vi "ObjectHandler.Main.vi"() -> ()   [LabVIEW 2016, in "ObjectHandler.lvclass"]
uses:
  ObjectHandler.lvclass
  Package Libraries/Message Queue/private/MessageQueue.MessageTypeDef.ctl
  ObjectHandler.lvclass/ObjectHandler.ctl
  ObjectHandler.ObjectMessage.ctl
  ObjectHandler.ObjectWType.ctl
  ObjectHandler.ObjectType.ctl
  ObjectHandler.ObjectMessageWCaller.ctl
  ObjectHandler.GetObjectWType.ctl
  Package ErrorHandling/ErrorHandling.lvclass/ErrorHandling.ctl
  Package ErrorHandling/ErrorHandling.checkForErrorAndHandle.vi
  Package ErrorHandling/ErrorHandling.GetErrorHandler.vi
  Package Libraries/StringFunctions/StringFunctions_ReplaceAllBlindSigns.vi
  <vilib>/dlg_ctls.llb/Space Constant.vi
  Package Libraries/TimingFunctions/TimingFunctions_getUtcTimestamp.vi
  <vilib>/Utility/error.llb/Trim Whitespace.vi
  <vilib>/Utility/error.llb/Search and Replace Pattern.vi
  Package ErrorHandling/ErrorHandling.addLastErrorToFile.vi
  Package ErrorHandling/ErrorHandling.lvclass
panel:
  out "ObjectNames":string[](array[string])
  out "LastCaller":string
  out "State":string
  out "RefreshTime":timestamp
  out "StartTime":timestamp
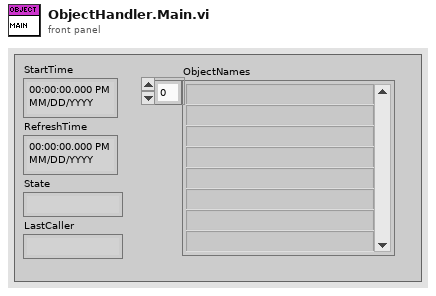
[diagram p1: front panel]
types:
  T1 = typedef "MessageQueue.MessageTypeDef.ctl" = cluster{"Message":string, "Data":variant}
  T2 = typedef "ObjectHandler.lvclass/ObjectHandler.ObjectMessage.ctl" = cluster{"Name":string, "ObjectWType":T3}
  T3 = typedef "ObjectHandler.lvclass/ObjectHandler.ObjectWType.ctl" = cluster{"ObjectType":T4, "Object":variant}
  T4 = typedef "ObjectHandler.lvclass/ObjectHandler.ObjectType.ctl" = enum16{"undefined", "ObjectHandler", "ViHandler", "ErrorHandler", "CentralStorage", "Hausmodell", "Sondenmodell", "Wärmepumpe", "Umgebung"}
  T5 = typedef "ObjectHandler.lvclass/ObjectHandler.ObjectMessageWCaller.ctl" = cluster{"Name":string, "ObjectWType":T3, "Caller":string}
  T6 = typedef "ObjectHandler.lvclass/ObjectHandler.GetObjectWType.ctl" = cluster{"Name":string, "Caller":string}
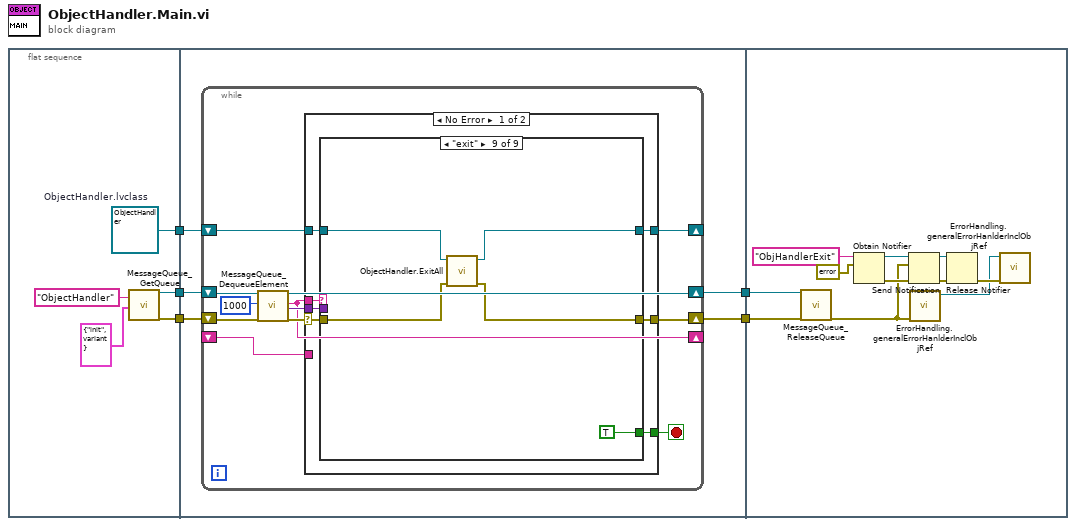
[diagram p0: block diagram]
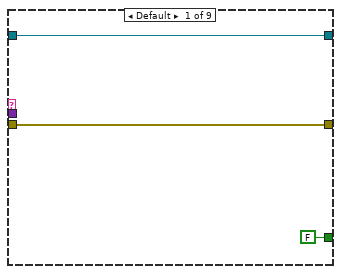
[diagram p2: hidden frame]
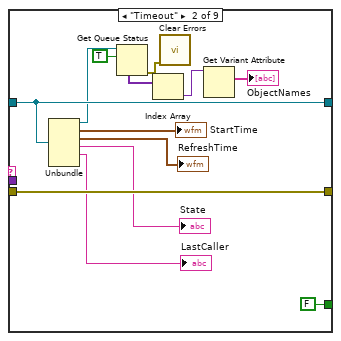
[diagram p3: hidden frame]
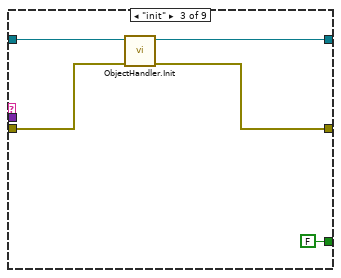
[diagram p4: hidden frame]
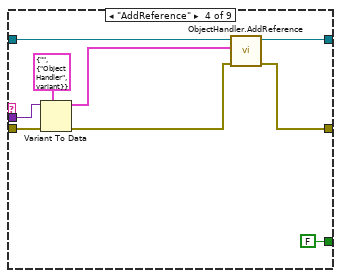
[diagram p5: hidden frame]
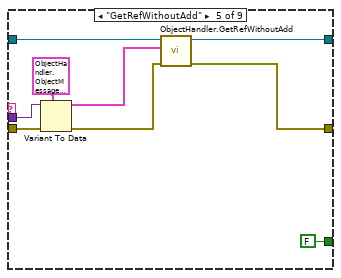
[diagram p6: hidden frame]
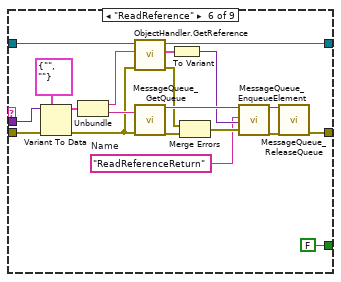
[diagram p7: hidden frame]
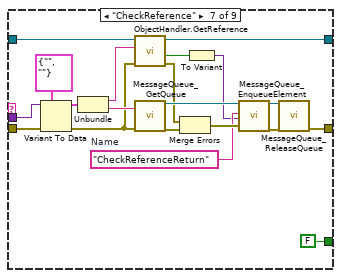
[diagram p8: hidden frame]
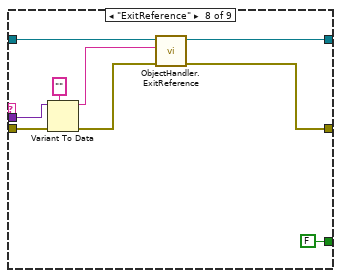
[diagram p9: hidden frame]
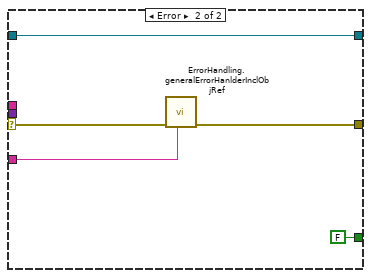
[diagram p10: hidden frame]
diagram:
  n1 = flat-sequence {
    tunnel: [w7] -> w5
    tunnel: [w9] -> w4
    tunnel: [w8] -> w3
    tunnel: w5 -> [w13]
    tunnel: w4 -> [w15]
    tunnel: w3 -> [w14]
    tunnel: [w12] -> w2
    tunnel: [w11] -> w1
    tunnel: w2 -> [w143]
    tunnel: w1 -> [w142]
    frame #0 {
      w7 = refnum<class "ObjectHandler.lvclass"> refnum  # ObjectHandler.lvclass
      n2 = call "MessageQueue_GetQueue.vi"("Name"="ObjectHandler", "OptionalInitValue"=T1 {"Message"="init", "Data"=variant}) -> ("QueueOut"=w9:refnum<queue>, "ErrorOut"=w8:errorcluster)  [unwired: 15 in, 1 out]
    }
    frame #1 {
      n3 = while {
        shift-right: [w22] -> _
        shift-left: w13 -> [w23]
        shift-right: [w18] -> w12
        shift-left: w14 -> [w27]
        shift-right: [w19] -> w11
        shift-left: w15 -> [w26]
        shift-right: [w17] -> _
        shift-left: _ -> [w16]
        stop <- w21 stop-if-true
        n4 = call "MessageQueue_DequeueElement.vi"("QueueIn"=w26, "Timeout"=1000, "ErrorIn"=w27) -> ("QueueOut"=w19:refnum<queue>, "Message"=w17:string, "Data"=w24:variant, "ErrorOut"=w25:errorcluster)  [unwired: 12 in, 1 out]
        n5 = case shown="No Error" w25 {
          selector: w25 -> [w32 w130]
          tunnel: w17 -> [w34 _]
          tunnel: w24 -> [w33 _]
          tunnel: w23 -> [w31 w132]
          tunnel: [w30 w132] -> w22
          tunnel: [w29 w129] -> w18
          tunnel: [w28 FALSE] -> w21
          tunnel: w16 -> [_ w128]
          frame No Error {
            n6 = case shown="\"exit\"" w34 {
              tunnel: w33 -> [_ _ _ w64 w73 w93 w113 w119 _]
              tunnel: w32 -> [w36 w50 w55 w63 w72 w92 w112 w120 w125]
              tunnel: w31 -> [w37 w48 w54 w62 w68 w90 w110 w122 w126]
              tunnel: [w37 w48 w53 w61 w67 w89 w109 w121 w124] -> w30
              tunnel: [w36 w50 w52 w59 w70 w79 w99 w115 w123] -> w29
              tunnel: [FALSE FALSE FALSE FALSE FALSE FALSE FALSE FALSE TRUE] -> w28
              frame Default {
              }
              frame "Timeout" {
                n7 = Unbundle(w48) -> (w43:refnum<queue>, →"StartTime":timestamp, →"RefreshTime":timestamp, →"State":string, →"LastCaller":string)  [unwired: 1 out]
                n8 = Get Queue Status(queue=w43, return elements? (F)=TRUE) -> (error out=w38:errorcluster, elements=w41:variant[])  [unwired: 1 in, 6 out]
                n9 = Index Array(array=w41) -> (element=w40:variant)  [unwired: 1 in]
                n10 = call <vilib>:"Clear Errors.vi"("error in (no error)"=w38) -> ()  [unwired: 5 in, 2 out]
                n11 = Get Variant Attribute(Variant=w40) -> (names=→"ObjectNames":string[])  [unwired: 3 in, 3 out]
              }
              frame "init" {
                n12 = call "ObjectHandler.Init.vi"("error in (no error)"=w55, "ObjectHandler in"=w54) -> ("error out"=w52:errorcluster, "ObjectHandler out"=w53:refnum<class "ObjectHandler.lvclass">)  [unwired: 8 in]
              }
              frame "AddReference" {
                n13 = Variant To Data(error in=w63, type=T2 {"Name"="", "ObjectWType"={"ObjectType"=enum."ObjectHandler", "Object"=variant(refnum<data-value> refnum)}} ("ObjectMessage"), Variant=w64) -> (data=w56:T2, error out=w60:errorcluster)
                n14 = call "ObjectHandler.AddReference.vi"("error in (no error)"=w60, "ObjectMessage"=w56, "ObjectHandler in"=w62) -> ("error out"=w59:errorcluster, "ObjectHandler out"=w61:refnum<class "ObjectHandler.lvclass">)  [unwired: 7 in]
              }
              frame "GetRefWithoutAdd" {
                n15 = Variant To Data(error in=w72, type=T5 {"Name"="", "ObjectWType"={"ObjectType"=enum."ObjectHandler", "Object"=variant(refnum<data-value> refnum)}, "Caller"=""} ("ObjectMessage"), Variant=w73) -> (data=w65:T5, error out=w69:errorcluster)
                n16 = call "ObjectHandler.GetRefWithoutAdd.vi"("error in (no error)"=w69, "data"=w65, "ObjectHandler in"=w68) -> ("error out"=w70:errorcluster, "ObjectHandler out"=w67:refnum<class "ObjectHandler.lvclass">)  [unwired: 7 in]
              }
              frame "ReadReference" {
                w74 = "ReadReferenceReturn"  # Name
                n17 = Variant To Data(error in=w92, type=T6 {"Name"="", "Caller"=""} ("GetRefInput"), Variant=w93) -> (data=w87:T6, error out=w84:errorcluster)
                n18 = Unbundle(w87) -> ("Name"=w86:string, "Caller"=w85:string)
                n19 = call "ObjectHandler.GetReference.vi"("error in (no error)"=w84, "Name"=w86, "ObjectHandler in"=w90) -> ("error out"=w82:errorcluster, "ObjectWType"=w76:T3, "ObjectHandler out"=w89:refnum<class "ObjectHandler.lvclass">)  [unwired: 5 in, 1 out]
                n20 = call "MessageQueue_GetQueue.vi"("Name"=w85, "ErrorIn"=w84) -> ("QueueOut"=w83:refnum<queue>, "ErrorOut"=w80:errorcluster)  [unwired: 15 in, 1 out]
                n21 = To Variant(anything=w76) -> (Variant=w75:variant)
                n22 = Merge Errors(w82, w80) -> (w81:errorcluster)
                n23 = call "MessageQueue_EnqueueElement.vi"("QueueIn"=w83, "Message"=w74, "Data"=w75, "ErrorIn"=w81) -> ("QueueOut"=w77:refnum<queue>, "ErrorOut"=w78:errorcluster)  [unwired: 14 in]
                n24 = call "MessageQueue_ReleaseQueue.vi"("QueueIn"=w77, "ErrorIn"=w78) -> ("ErrorOut"=w79:errorcluster)  [unwired: 15 in, 2 out]
              }
              frame "CheckReference" {
                w96 = "CheckReferenceReturn"  # Name
                n25 = Variant To Data(error in=w112, type=T6 {"Name"="", "Caller"=""} ("GetRefInput"), Variant=w113) -> (data=w107:T6, error out=w104:errorcluster)
                n26 = Unbundle(w107) -> ("Name"=w106:string, "Caller"=w105:string)
                n27 = call "ObjectHandler.GetReference.vi"("error in (no error)"=w104, "Name"=w106, "ObjectHandler in"=w110) -> ("error out"=w102:errorcluster, "Found?"=w95:bool, "ObjectHandler out"=w109:refnum<class "ObjectHandler.lvclass">)  [unwired: 5 in, 1 out]
                n28 = call "MessageQueue_GetQueue.vi"("Name"=w105, "ErrorIn"=w104) -> ("QueueOut"=w103:refnum<queue>, "ErrorOut"=w100:errorcluster)  [unwired: 15 in, 1 out]
                n29 = Merge Errors(w102, w100) -> (w101:errorcluster)
                n30 = To Variant(anything=w95) -> (Variant=w94:variant)
                n31 = call "MessageQueue_EnqueueElement.vi"("QueueIn"=w103, "Message"=w96, "Data"=w94, "ErrorIn"=w101) -> ("QueueOut"=w97:refnum<queue>, "ErrorOut"=w98:errorcluster)  [unwired: 14 in]
                n32 = call "MessageQueue_ReleaseQueue.vi"("QueueIn"=w97, "ErrorIn"=w98) -> ("ErrorOut"=w99:errorcluster)  [unwired: 15 in, 2 out]
              }
              frame "ExitReference" {
                n33 = Variant To Data(error in=w120, type="", Variant=w119) -> (data=w117:string, error out=w116:errorcluster)
                n34 = call "ObjectHandler.ExitReference.vi"("error in (no error)"=w116, "Name"=w117, "ObjectHandler in"=w122) -> ("error out"=w115:errorcluster, "ObjectHandler out"=w121:refnum<class "ObjectHandler.lvclass">)  [unwired: 7 in]
              }
              frame "exit" {
                n35 = call "ObjectHandler.ExitAll.vi"("error in"=w125, "ObjectHandler in"=w126) -> ("error out"=w123:errorcluster, "ObjectHandler out"=w124:refnum<class "ObjectHandler.lvclass">)  [unwired: 8 in]
              }
            }
          }
          frame Error {
            n36 = call "ErrorHandling.generalErrorHanlderInclObjRef.vi"("LastCommand(optional)"=w128, "error in"=w130) -> ("error out"=w129:errorcluster)  [unwired: 7 in, 2 out]
          }
        }
      }
    }
    frame #2 {
      n37 = call "MessageQueue_ReleaseQueue.vi"("QueueIn"=w142, "ErrorIn"=w143) -> ("ErrorOut"=w134:errorcluster)  [unwired: 15 in, 2 out]
      n38 = Obtain Notifier(name (unnamed)="ObjHandlerExit", notification data type=errorcluster {"status"=FALSE, "code"=0, "source"=""} ("ErrorOut")) -> (notifier out=w139:refnum<notifier>, error out=w140:errorcluster)  [unwired: 2 in, 1 out]
      n39 = Send Notification(notification=w134, notifier=w139, error in (no error)=w140) -> (notifier out=w137:refnum<notifier>, error out=w138:errorcluster)
      n40 = call "ErrorHandling.generalErrorHanlderInclObjRef.vi"("error in"=w134) -> ("ErrorHandling out"=w133:refnum<data-value>)  [unwired: 8 in, 2 out]
      n41 = Release Notifier(notifier=w137, error in (no error)=w138) -> (error out=w135:errorcluster)  [unwired: 1 in, 2 out]
      n42 = call "ErrorHandling.generalErrorHanlderInclObjRef.vi"("error in"=w135, "ErrorHandling(optional)"=w133) -> ()  [unwired: 7 in, 3 out]
    }
  }
